vi "Upgrade Component Dependencies.vi"(0 "VIPM In":refnum<class "VIP.lvclass">, 11 "error in (no error)":errorcluster) -> (4 "VIPM Out":refnum<class "VIP.lvclass">, 15 "error out":errorcluster)   [LabVIEW 2017, in "CL_G3_VIComponentBuilder.lvlib" / "VIP.lvclass"]
doc: "Upgrades this VI Packages build spec to list the most recent version of all of its dependencies. Adds a release note to indicate which dependencies were upgraded from what version to what version."
uses:
  VIP.lvclass
  C:/Tool Chain Support/Software Module Builder/Source/Exports/Exports/Export.lvclass
  Exports/Export.lvclass/Export.ctl
  <vilib>/Utility/error.llb/whitespace.ctl
  Exports/Accessors/Read Exported Build Specification Path.vi
  <vilib>/xml/Close Reference(Node).vi
  <vilib>/xml/Close Reference(NdList).vi
  Exports/Export.lvclass
  <vilib>/xml/NI_XML.lvlib
  <resource>/objmgr/DOMUserDefRef.rc
  VIPM Utilities/CL_G3_VIPMUtilities.lvlib
  CL_G3_VIComponentBuilder.lvlib
panel:
  out "Upgrade Information":T1(array[cluster])
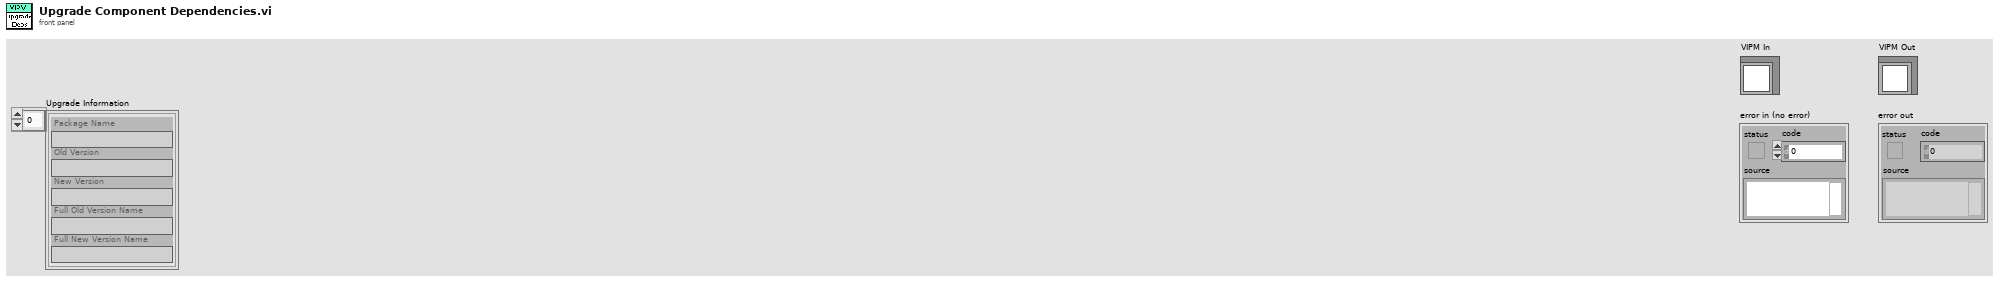
[diagram p1: front panel]
types:
  T1 = cluster{"Package Name":string, "Old Version":string, "New Version":string, "Full Old Version Name":string, "Full New Version Name":string}[]
  T2 = cluster{"Package Name":string, "Old Version":string, "New Version":string, "Full Old Version Name":string, "Full New Version Name":string}
  T3 = typedef "whitespace.ctl" = u16
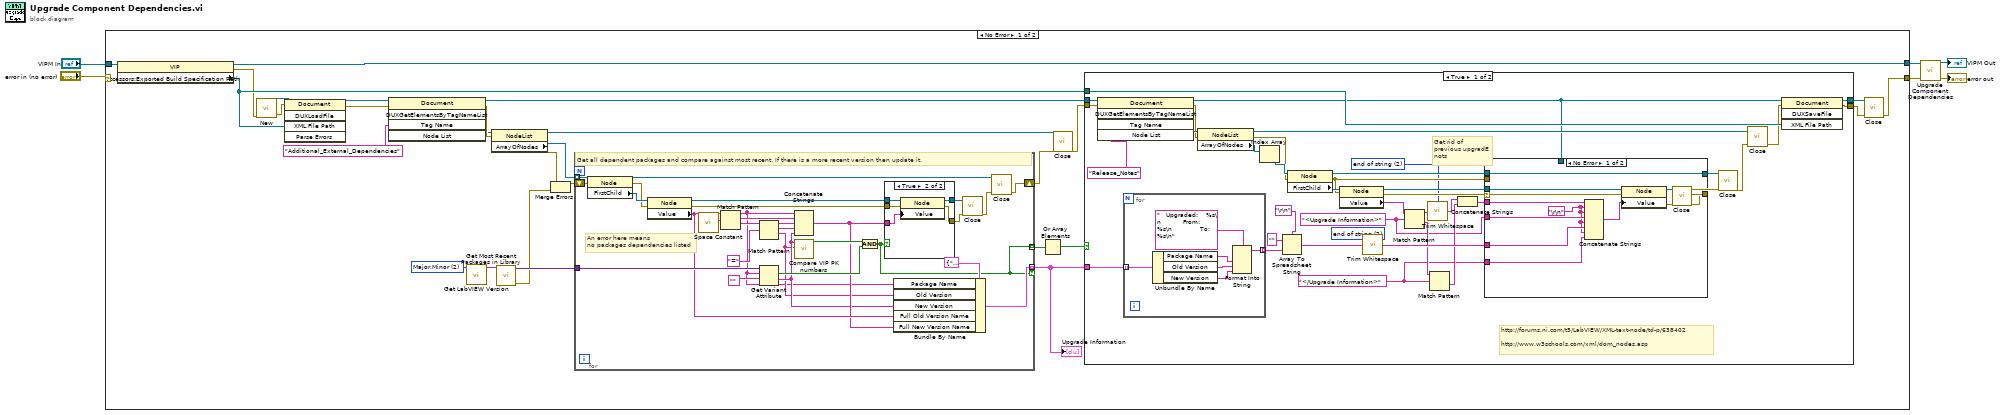
[diagram p0: block diagram]
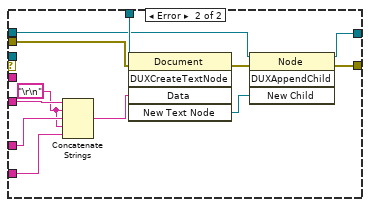
[diagram p2: hidden frame]
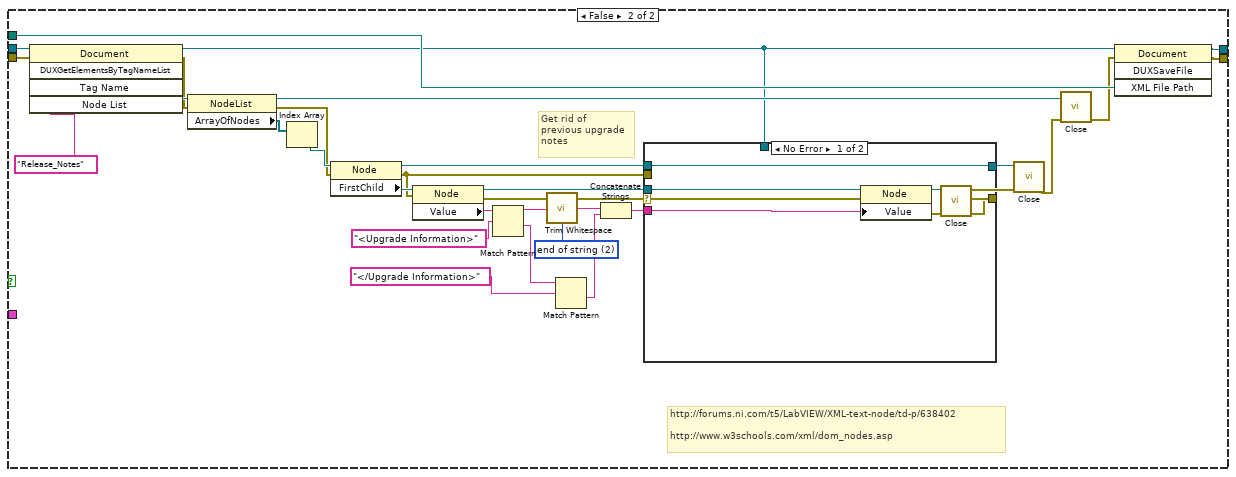
[diagram p3: hidden frame]
diagram:
  n1 = case shown="No Error" "error in (no error)" {
    selector: "error in (no error)" -> [_ w179]
    tunnel: "VIPM In" -> [w16 w180]
    tunnel: [w14 w180] -> w4
    tunnel: [w13 w179] -> w1
    frame No Error {
      w10 = u16 2 items=["Major"=1, "Major.Minor"=2, "Major.Minor.Fix"=3] ("Type Of LabVIEW Version Descriptor")
      n2 = property class="VIP"(reference=w16) -> (reference out=w14:refnum<class "VIP.lvclass">, error out=w12:errorcluster, "Accessors:Exported Build Specification Path"=w15:path)  [unwired: 1 in]
      n3 = call <vilib>:"New.vi"("error in (no error)"=w12) -> ("error out"=w32:errorcluster, "DOM document out"=w31:refnum<k20>)  [unwired: 7 in]
      n4 = invoke class="Document" method="DUXLoadFile"(reference=w31, error in=w32, "XML File Path"=w15) -> (reference out=w33:refnum<k20>, error out=w25:errorcluster)  [unwired: 2 in, 3 out]
      n5 = invoke class="Document" method="DUXGetElementsByTagNameList"(reference=w33, error in=w25, "Tag Name"="Additional_External_Dependencies") -> (reference out=w20:refnum<k20>, error out=w28:errorcluster, "Node List"=w26:refnum<k20>)  [unwired: 2 in, 2 out]
      n6 = call "Get LabVIEW Version.vi"("Type Of LabVIEW Version Descriptor"=w10) -> ("LabVIEW Version"=w11:string)  [unwired: 13 in, 1 out]
      n7 = property class="NodeList"(reference=w26, error in=w28) -> (reference out=w29:refnum<k20>, error out=w8:errorcluster, "ArrayOfNodes"=w27:refnum<k20>[])
      n8 = call "Get Most Recent Packages in Library.vi"("LabVIEW Version (14.0)"=w11) -> ("error out"=w9:errorcluster, "Varriant Attibute Table of newest Packages in Library"=w24:variant)  [unwired: 8 in, 1 out]
      n9 = Merge Errors(w8, w9) -> (w7:errorcluster)
      n10 = for {
        tunnel: w27 -> [w171] mode=indexing
        shift-right: [w165] -> w30
        shift-left: w7 -> [w169]
        tunnel: w24 -> [w161]
        tunnel: [w149] -> w19 mode=indexing if=w146
        tunnel: [w146] -> w21 mode=indexing
        # "An error here means\nno packages dependencies listed"
        # "Get all dependent packages and compare against most recent. If there is a more recent version then update it."
        n11 = property class="Node"(reference=w171, error in=w169) -> (reference out=w167:refnum<k20>, error out=w168:errorcluster, "FirstChild"=w170:refnum<k20>)
        n12 = property class="Node"(reference=w170, error in=w168) -> (reference out=w163:refnum<k20>, error out=w152:errorcluster, "Value"=w148:string)
        n13 = call <vilib>:"Space Constant.vi"() -> ("String"=w164:string)
        n14 = Match Pattern(string=w148, regular expression=w164) -> (before substring=w143:string, match substring=w155:string, after substring=w156:string)  [unwired: 1 in, 1 out]
        n15 = Match Pattern(string=w156, regular expression="=") -> (before substring=w157:string, match substring=w158:string, after substring=w144:string)  [unwired: 1 in, 1 out]
        n16 = Get Variant Attribute(Variant=w161, name=w143, default value (empty Variant)="") -> (found=w154:bool, value=w145:string)  [unwired: 1 in, 2 out]
        n17 = Concatenate Strings(w143, w155, w157, w158, w145) -> (w147:string)
        n18 = call "Compare VIP PK numbers.vi"("Y (#.#.#.#)"=w144, "X (#.#.#.#)"=w145) -> ("X>Y"=w153:bool)  [unwired: 8 in, 1 out]
        n19 = And(x=w153, y=w154) -> (x .and. y?=w146:bool)
        n20 = case shown="True" w146 {
          tunnel: w163 -> [w173 w178]
          tunnel: [w173 w177] -> w162
          tunnel: w147 -> [_ w176]
          tunnel: w152 -> [w172 w175]
          tunnel: [w172 w174] -> w151
          frame False {
          }
          frame True {
            n21 = property class="Node"(reference=w178, error in=w175, "Value"=w176) -> (reference out=w177:refnum<k20>, error out=w174:errorcluster)
          }
        }
        n22 = Bundle By Name(cluster=T2 {"Package Name"="", "Old Version"="", "New Version"="", "Full Old Version Name"="", "Full New Version Name"=""}, "Package Name"=w143, "Old Version"=w144, "New Version"=w145, "Full Old Version Name"=w148, "Full New Version Name"=w147) -> (w149:T2)
        n23 = call-poly <vilib>:"Close.vi"("error in (no error)"=w151, "node"=w162) -> ("error out"=w166:errorcluster)  [unwired: 7 in]
        n24 = call-poly <vilib>:"Close.vi"("error in (no error)"=w166, "node"=w167) -> ("error out"=w165:errorcluster)  [unwired: 7 in]
      }
      "Upgrade Information" <- w19
      n25 = Or Array Elements(Boolean array=w21) -> (logical OR=w17:bool)
      n26 = call-poly <vilib>:"Close.vi"("error in (no error)"=w30, "node list"=w29) -> ("error out"=w18:errorcluster)  [unwired: 7 in]
      n27 = case shown="True" w17 {
        tunnel: [w72 w133] -> w23
        tunnel: [w71 w132] -> w22
        tunnel: w15 -> [w70 w131]
        tunnel: w20 -> [w69 w130]
        tunnel: w19 -> [w66 _]
        tunnel: w18 -> [w63 w126]
        frame True {
          w37 = T3 2 items=["both", "start of string", "end of string"] ("location (both)")
          w46 = T3 2 items=["both", "start of string", "end of string"] ("location (both)")
          w38 = "</Upgrade Information>" ("format string")
          w39 = "<Upgrade Information>" ("format string")
          # "Get rid of \nprevious upgradE\nnots"
          # "http://forums.ni.com/t5/LabVIEW/XML-text-node/td-p/638402\n\nhttp://www.w3schools.com/xml/dom_nodes.asp"
          n28 = invoke class="Document" method="DUXGetElementsByTagNameList"(reference=w69, error in=w63, "Tag Name"="Release_Notes") -> (reference out=w51:refnum<k20>, error out=w64:errorcluster, "Node List"=w67:refnum<k20>)  [unwired: 2 in, 2 out]
          n29 = for {
            tunnel: w66 -> [w102] mode=indexing
            tunnel: [w97] -> w65 mode=indexing
            n30 = Unbundle By Name(w102) -> ("Package Name"=w100:string, "Old Version"=w99:string, "New Version"=w98:string)
            n31 = Format Into String(format string="   Upgraded:    %s\n           From:    %s\n              To:     %s\n", w100, w99, w98) -> (resulting string=w97:string)  [unwired: 2 in, 1 out]
          }
          n32 = property class="NodeList"(reference=w67, error in=w64) -> (reference out=w57:refnum<k20>, error out=w58:errorcluster, "ArrayOfNodes"=w62:refnum<k20>[])
          n33 = Index Array(array=w62) -> (element=w61:refnum<k20>)  [unwired: 1 in]
          n34 = Array To Spreadsheet String(delimiter (Tab)="\r\n", array=w65, 3:"" ("format string")) -> (spreadsheet string=w45:string)
          n35 = property class="Node"(reference=w61, error in=w58) -> (reference out=w49:refnum<k20>, error out=w50:errorcluster, "FirstChild"=w60:refnum<k20>)
          n36 = property class="Node"(reference=w60, error in=w50) -> (reference out=w59:refnum<k20>, error out=w52:errorcluster, "Value"=w43:string)
          n37 = call <vilib>:"Trim Whitespace.vi"("string"=w45, "location (both)"=w46) -> ("trimmed string"=w44:string)
          n38 = Match Pattern(string=w43, regular expression=w39) -> (before substring=w36:string, after substring=w42:string)  [unwired: 1 in, 2 out]
          n39 = call <vilib>:"Trim Whitespace.vi"("string"=w36, "location (both)"=w37) -> ("trimmed string"=w35:string)
          n40 = Match Pattern(string=w42, regular expression=w38) -> (after substring=w41:string)  [unwired: 1 in, 3 out]
          n41 = Concatenate Strings(w35, w41) -> (w40:string)
          n42 = case shown="No Error" w52 {
            selector: w52 -> [w83 _]
            tunnel: [w80 w91] -> w48
            tunnel: w59 -> [w84 _]
            tunnel: w51 -> [_ w96]
            tunnel: w50 -> [_ w95]
            tunnel: w49 -> [w79 w94]
            tunnel: [w79 w90] -> w47
            tunnel: w38 -> [w78 w87]
            tunnel: w44 -> [w77 w88]
            tunnel: w40 -> [w75 _]
            tunnel: w39 -> [w74 w89]
            frame No Error {
              w73 = "\r\n"
              n43 = Concatenate Strings(w75, w73, w73, w74, w73, w77, w73, w78) -> (w76:string)
              n44 = property class="Node"(reference=w84, error in=w83, "Value"=w76) -> (reference out=w82:refnum<k20>, error out=w81:errorcluster)
              n45 = call-poly <vilib>:"Close.vi"("error in (no error)"=w81, "node"=w82) -> ("error out"=w80:errorcluster)  [unwired: 7 in]
            }
            frame Error {
              w85 = "\r\n"
              n46 = Concatenate Strings(w89, w85, w88, w85, w87) -> (w86:string)
              n47 = invoke class="Document" method="DUXCreateTextNode"(reference=w96, error in=w95, "Data"=w86) -> (error out=w92:errorcluster, "New Text Node"=w93:refnum<k20>)  [unwired: 2 in, 3 out]
              n48 = invoke class="Node" method="DUXAppendChild"(reference=w94, error in=w92, "New Child"=w93) -> (reference out=w90:refnum<k20>, error out=w91:errorcluster)  [unwired: 1 in, 2 out]
            }
          }
          n49 = call-poly <vilib>:"Close.vi"("error in (no error)"=w48, "node"=w47) -> ("error out"=w56:errorcluster)  [unwired: 7 in]
          n50 = call-poly <vilib>:"Close.vi"("error in (no error)"=w56, "node list"=w57) -> ("error out"=w55:errorcluster)  [unwired: 7 in]
          n51 = invoke class="Document" method="DUXSaveFile"(reference=w51, error in=w55, "XML File Path"=w70) -> (reference out=w72:refnum<k20>, error out=w71:errorcluster)  [unwired: 1 in, 2 out]
        }
        frame False {
          w105 = T3 2 items=["both", "start of string", "end of string"] ("location (both)")
          # "Get rid of \nprevious upgrade\nnotes"
          # "http://forums.ni.com/t5/LabVIEW/XML-text-node/td-p/638402\n\nhttp://www.w3schools.com/xml/dom_nodes.asp"
          n52 = invoke class="Document" method="DUXGetElementsByTagNameList"(reference=w130, error in=w126, "Tag Name"="Release_Notes") -> (reference out=w116:refnum<k20>, error out=w127:errorcluster, "Node List"=w128:refnum<k20>)  [unwired: 2 in, 2 out]
          n53 = property class="NodeList"(reference=w128, error in=w127) -> (reference out=w120:refnum<k20>, error out=w121:errorcluster, "ArrayOfNodes"=w125:refnum<k20>[])
          n54 = Index Array(array=w125) -> (element=w124:refnum<k20>)  [unwired: 1 in]
          n55 = property class="Node"(reference=w124, error in=w121) -> (reference out=w114:refnum<k20>, error out=w115:errorcluster, "FirstChild"=w123:refnum<k20>)
          n56 = property class="Node"(reference=w123, error in=w115) -> (reference out=w122:refnum<k20>, error out=w117:errorcluster, "Value"=w111:string)
          n57 = Match Pattern(string=w111, regular expression="<Upgrade Information>" ("format string")) -> (before substring=w104:string, after substring=w110:string)  [unwired: 1 in, 2 out]
          n58 = call <vilib>:"Trim Whitespace.vi"("string"=w104, "location (both)"=w105) -> ("trimmed string"=w103:string)
          n59 = Match Pattern(string=w110, regular expression="</Upgrade Information>" ("format string")) -> (after substring=w109:string)  [unwired: 1 in, 3 out]
          n60 = Concatenate Strings(w103, w109) -> (w108:string)
          n61 = case shown="No Error" w117 {
            selector: w117 -> [w139 _]
            tunnel: [w136 w141] -> w113
            tunnel: w122 -> [w140 _]
            tunnel: w116 -> [_ _]
            tunnel: w115 -> [_ w141]
            tunnel: w114 -> [w135 w142]
            tunnel: [w135 w142] -> w112
            tunnel: w108 -> [w134 _]
            frame No Error {
              n62 = property class="Node"(reference=w140, error in=w139, "Value"=w134) -> (reference out=w138:refnum<k20>, error out=w137:errorcluster)
              n63 = call-poly <vilib>:"Close.vi"("error in (no error)"=w137, "node"=w138) -> ("error out"=w136:errorcluster)  [unwired: 7 in]
            }
            frame Error {
              # "node doesn't exist so don't create it."
            }
          }
          n64 = call-poly <vilib>:"Close.vi"("error in (no error)"=w113, "node"=w112) -> ("error out"=w119:errorcluster)  [unwired: 7 in]
          n65 = call-poly <vilib>:"Close.vi"("error in (no error)"=w119, "node list"=w120) -> ("error out"=w118:errorcluster)  [unwired: 7 in]
          n66 = invoke class="Document" method="DUXSaveFile"(reference=w116, error in=w118, "XML File Path"=w131) -> (reference out=w133:refnum<k20>, error out=w132:errorcluster)  [unwired: 1 in, 2 out]
        }
      }
      n67 = call-poly <vilib>:"Close.vi"("error in (no error)"=w22, "node"=w23) -> ("error out"=w13:errorcluster)  [unwired: 7 in]
    }
    frame Error {
    }
  }
  n68 = call-parent "Upgrade Component Dependencies.vi"("Export In"=w4, "error in (no error)"=w1) -> ("Export Out"=→"VIPM Out":refnum<class "VIP.lvclass">, "error out"=→"error out":errorcluster)  [unwired: 12 in]
